vi "Display Tree Item.vi"(8 "error in (no error)":errorcluster, 10 "Tag":string, 11 "Application Data in":T1) -> (0 "error out":errorcluster, 3 "Application Data out":T1)   [LabVIEW 2017, in "DSF Data Viewer.lvlib"]
uses:
  DSF Data Viewer.lvlib
  Application Data.ctl
  Builds/Data Sharing Framework/Current/Core/DSF Core.lvlibp/Engine/Classes/Framework/Framework.lvclass
  <vilib>/NI/Memory Manager/Classes/Pointer/Pointer.lvclass
  Buffer Reader/Buffer Data.ctl
  Builds/Data Sharing Framework/Current/Core/DSF Core.lvlibp/Engine/Classes/Buffer/Buffer.lvclass
  Builds/Data Sharing Framework/Current/Core/DSF Core.lvlibp/DSF Configuration API/Configuration Session.lvclass
  Builds/Data Sharing Framework/Current/Core/DSF Core.lvlibp/DSF Configuration API/Public/Read Item/Read Group.vi
  Builds/Data Sharing Framework/Current/Core/DSF Core.lvlibp/DSF Configuration API/Public/Read Item/Read Channel.vi
  Builds/Data Sharing Framework/Current/Core/DSF Core.lvlibp/DSF Configuration API/Public/Read Item/Read Transfer.vi
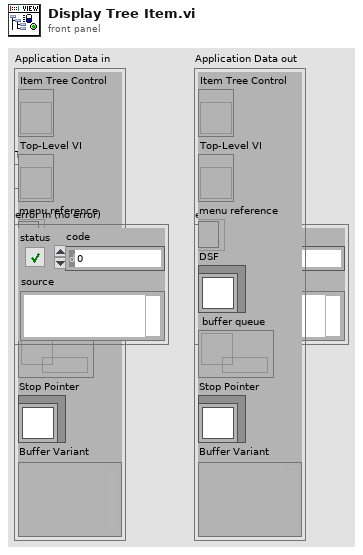
[diagram p1: front panel]
types:
  T1 = typedef "DSF Data Viewer.lvlib/Application Data.ctl" = cluster{"Item Tree Control":refnum<vi>, "Top-Level VI":refnum<vi>, "menu reference":refnum<k9>, "DSF":refnum<class "Framework.lvclass">, "buffer queue":refnum<queue>, "Stop Pointer":refnum<class "Pointer.lvclass">, "Buffer Variant":variant}
  T2 = typedef "DSF Data Viewer.lvlib/Buffer Data.ctl" = cluster{"Buffer":refnum<class "Buffer.lvclass">, "decimation":u64}
  T3 = typedef "DSF Data Viewer.lvlib/Tree Item Type.ctl" = enum16{"Framework", "Plugin Group", "Plugin", "Group", "Transfer", "Buffer", "Channel"}
  T4 = typedef "DSF Core.lvlibp/DSF Group Info.ctl" = cluster{"direction":T5, "timing":T6, "transfer ids":string[], "settings id":string, "thread":i32}
  T5 = typedef "DSF Core.lvlibp/DSF Direction.ctl" = enum8{"Tx", "Rx"}
  T6 = typedef "DSF Core.lvlibp/DSF Timing Info.ctl" = cluster{"priority":u64, "decimation":u64, "offset":u64}
  T7 = typedef "DSF Core.lvlibp/DSF Transfer Info.ctl" = cluster{"byte order":T8, "channel ids":string[], "settings id":string}
  T8 = typedef "DSF Core.lvlibp/DSF Byte Order.ctl" = enum8{"big-endian", "little-endian"}
  T9 = typedef "DSF Core.lvlibp/DSF Channel Info.ctl" = cluster{"string buffer offset":u64, "string data type":T10, "engine data type":T10, "settings id":string}
  T10 = typedef "DSF Core.lvlibp/DSF Data Type.ctl" = enum8{"Bool", "SGL", "DBL", "I8", "I16", "I32", "I64", "U8", "U16", "U32", "U64"}
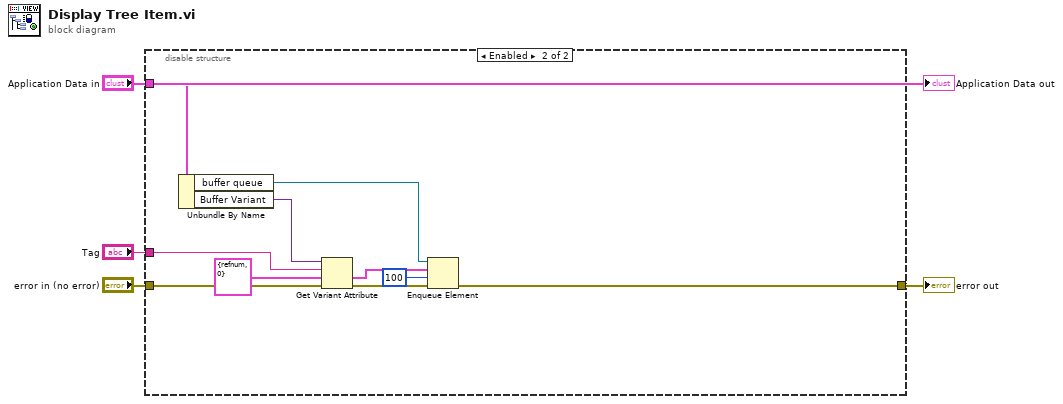
[diagram p0: block diagram]
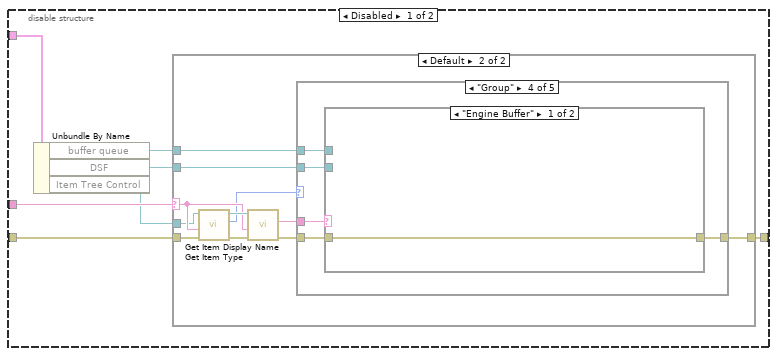
[diagram p2: hidden frame]
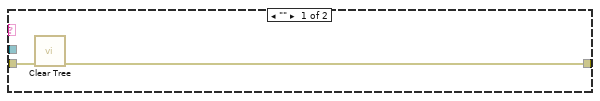
[diagram p3: hidden frame]
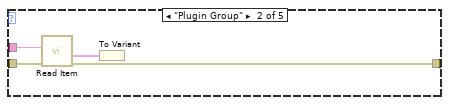
[diagram p5: hidden frame]
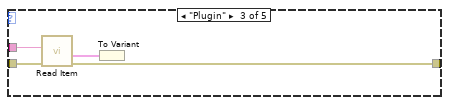
[diagram p6: hidden frame]
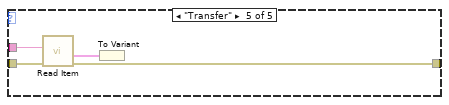
[diagram p8: hidden frame]
diagram:
  n1 = disable-structure shown="Enabled" {
    disable-tunnel: "Tag" -> [w11 w51]
    disable-tunnel: "Application Data in" -> [w10 w54]
    disable-tunnel: "error in (no error)" -> [w9 w52]
    disable-tunnel: [w8 w45] -> w1
    frame Disabled {
      n2 = Unbundle By Name(w10) -> ("buffer queue"=w5:refnum<queue>, "DSF"=w6:refnum<class "Framework.lvclass">, "Item Tree Control"=w7:refnum<vi>)
      n3 = case shown="Default" w11 {
        selector: w11 -> [_ w20]
        tunnel: w6 -> [_ w19]
        tunnel: w7 -> [_ w18]
        tunnel: w9 -> [w13 w17]
        tunnel: [w12 w14] -> w8
        tunnel: w5 -> [_ w15]
        frame "" {
          n4 = call "Clear Tree.vi"("error in (no error)"=w13) -> ("error out"=w12:errorcluster)  [unwired: 10 in]
        }
        frame Default {
          n5 = call "Get Item Type.vi"("error in (no error)"=w17, "Tag"=w20, "TreeControl in"=w18) -> ("error out"=w23:errorcluster, "Item Type"=w16:T3, "TreeControl out"=w22:refnum<vi>)  [unwired: 6 in]
          n6 = call "Get Item Display Name.vi"("error in (no error)"=w23, "Tag"=w20, "TreeControl in"=w22) -> ("error out"=w24:errorcluster, "display name"=w21:string)  [unwired: 6 in, 1 out]
          n7 = case shown="\"Group\"" w16 {
            tunnel: w21 -> [_ w26 w30 w38 w41]
            tunnel: [w25 w28 w31 w34 w42] -> w14
            tunnel: w24 -> [w25 w27 w32 w35 w43]
            tunnel: w19 -> [_ _ _ w37 _]
            tunnel: w15 -> [_ _ _ w36 _]
            frame "Framework" {
            }
            frame "Plugin Group" {
              n8 = call-poly "Read Item.vi"("error in (no error)"=w27, "Group ID"=w26) -> ("error out"=w28:errorcluster, "value"=w29:T4)  [unwired: 6 in, 2 out]
              n9 = To Variant(anything=w29) -> ()  [unwired: 1 out]
            }
            frame "Plugin" {
              n10 = call-poly "Read Item.vi"("error in (no error)"=w32, "Transfer ID"=w30) -> ("error out"=w31:errorcluster, "value"=w33:T7)  [unwired: 6 in, 2 out]
              n11 = To Variant(anything=w33) -> ()  [unwired: 1 out]
            }
            frame "Group" {
              n12 = case shown="\"Engine Buffer\"" w38 {
                tunnel: w37 -> [_ _]
                tunnel: w36 -> [_ _]
                tunnel: w35 -> [w39 w40]
                tunnel: [w39 w40] -> w34
                frame "Engine Buffer" {
                }
                frame Default {
                }
              }
            }
            frame "Transfer" {
              n13 = call-poly "Read Item.vi"("error in (no error)"=w43, "Channel ID"=w41) -> ("error out"=w42:errorcluster, "value"=w44:T9)  [unwired: 6 in, 2 out]
              n14 = To Variant(anything=w44) -> ()  [unwired: 1 out]
            }
          }
        }
      }
    }
    frame Enabled {
      n15 = Unbundle By Name(w54) -> ("buffer queue"=w48:refnum<queue>, "Buffer Variant"=w53:variant)
      n16 = Get Variant Attribute(Variant=w53, name=w51, default value (empty Variant)=T2 {"Buffer"=refnum, "decimation"=0} ("Buffer data"), error in=w52) -> (value=w46:T2, error out=w49:errorcluster)  [unwired: 2 out]
      n17 = Enqueue Element(queue=w48, element=w46, timeout in ms (-1)=100, error in (no error)=w49) -> (error out=w45:errorcluster)  [unwired: 2 out]
    }
  }
  "error out" <- w1
  "Application Data out" <- "Application Data in"
